vi "plotToString_MATLAB.vi"(4 "yAxisBounds":T1={"Min"={"Auto"=TRUE, "Value"=0.0}, "Max"={"Auto"=TRUE, "Value"=0.0}}, 5 "Interation number":i32, 6 "xAxisBounds":T1={"Min"={"Auto"=TRUE, "Value"=0.0}, "Max"={"Auto"=TRUE, "Value"=0.0}}, 7 "Error Bar Type":T5=enum."Standard Error", 8 "Plot Metadata":T3, 9 "Profile Number":string, 10 "Column2":dbl[](array[numeric]), 11 "Column1":dbl[](array[numeric])) -> (0 "Max Min array":dbl[][](array[numeric]), 1 "Error Bars?":bool, 2 "Data Directories":string[](array[string]), 3 "plotString":string)   [LabVIEW 2020]
uses:
  Anemometry/Anemometry Sub Vis/Data_plotting_vis/Error bar Type.ctl
  Anemometry/Anemometry Sub Vis/Data_plotting_vis/RFP_Plot_Metadata.ctl
  Anemometry/Anemometry Sub Vis/Data_plotting_vis/Error_bars_index.ctl
  Anemometry/Anemometry Sub Vis/Data_plotting_vis/gnuplotScriptComponents/minAndMax.ctl
  Anemometry/Anemometry Sub Vis/Data_plotting_vis/gnuplotScriptComponents/AutoManualNumber.ctl
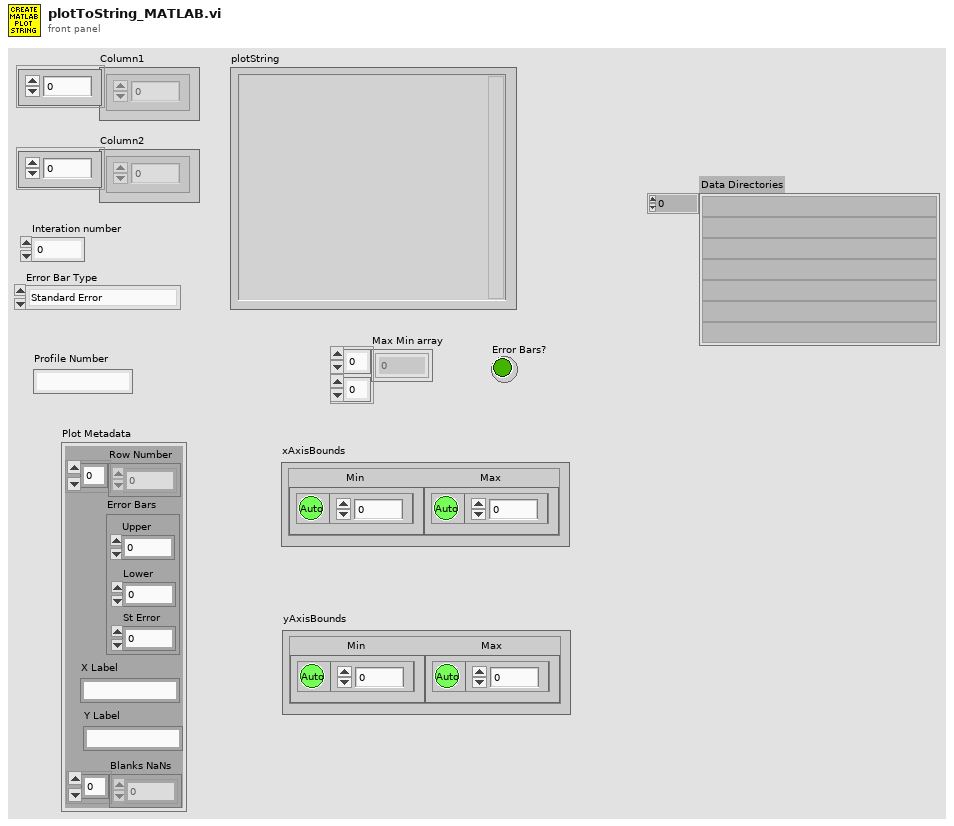
[diagram p1: front panel]
types:
  T1 = typedef "minAndMax.ctl" = cluster{"Min":T2, "Max":T2}
  T2 = typedef "AutoManualNumber.ctl" = cluster{"Auto":bool, "Value":dbl}
  T3 = typedef "RFP_Plot_Metadata.ctl" = cluster{"Row Number":i32[], "Error Bars":T4, "X Label":string, "Y Label":string, "Blanks NaNs":i32[]}
  T4 = typedef "Error_bars_index.ctl" = cluster{"Upper":i32, "Lower":i32, "St Error":i32}
  T5 = typedef "Error bar Type.ctl" = enum16{"None", "Standard Error", "Separate upper and lower"}
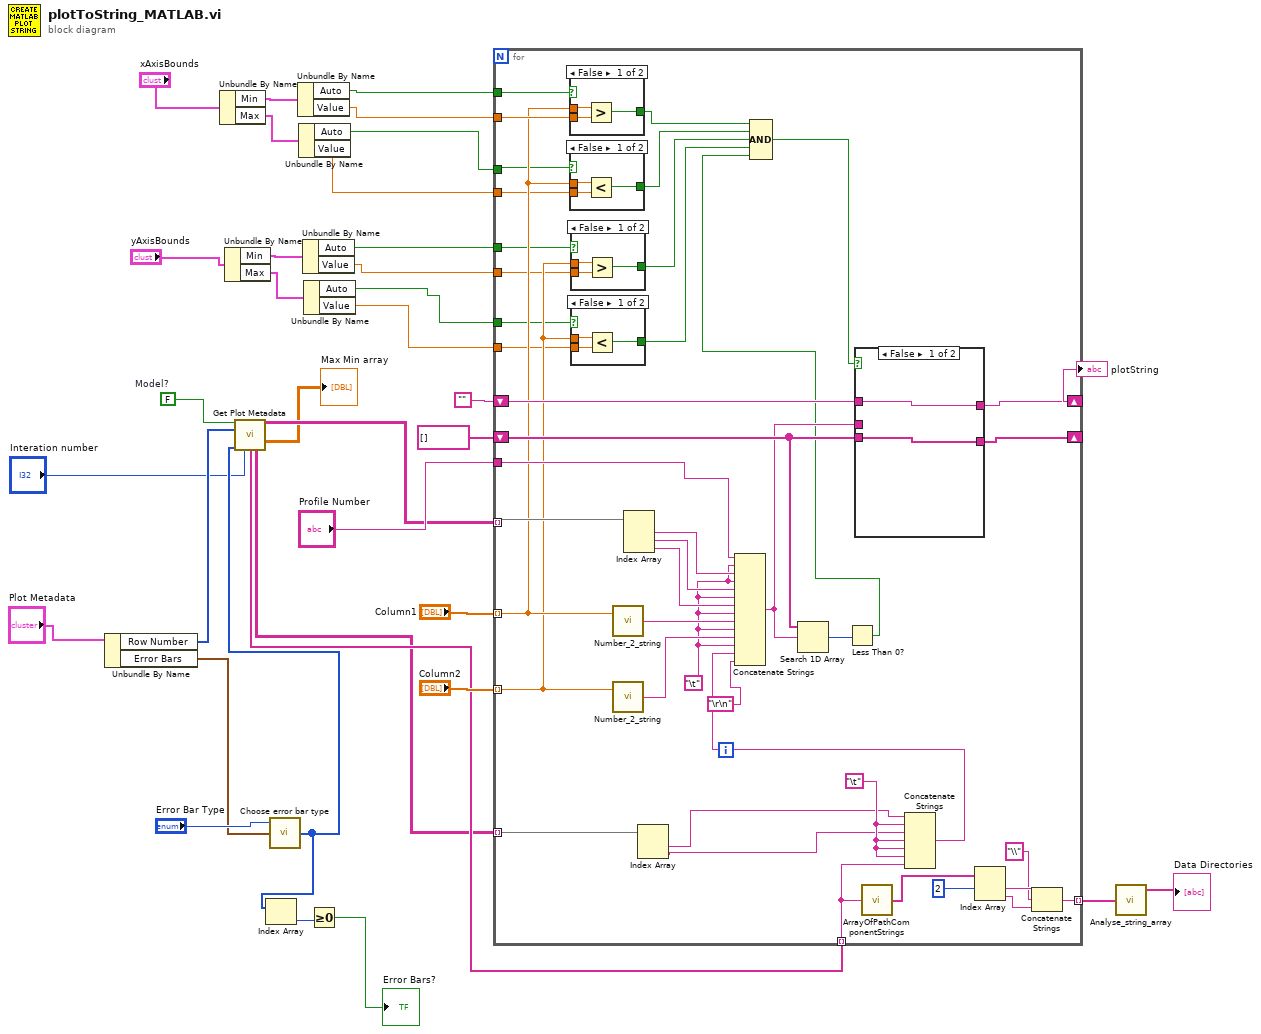
[diagram p0: block diagram]
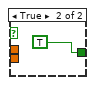
[diagram p2: hidden frame]
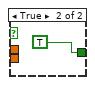
[diagram p3: hidden frame]
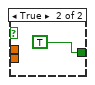
[diagram p4: hidden frame]
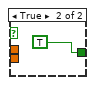
[diagram p5: hidden frame]
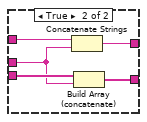
[diagram p6: hidden frame]
diagram:
  w25 = FALSE  # Model?
  n1 = Unbundle By Name("Plot Metadata") -> ("Row Number"=w28:i32[], "Error Bars"=w23:T4)
  n2 = Unbundle By Name("xAxisBounds") -> ("Min"=w16:T2, "Max"=w14:T2)
  n3 = Unbundle By Name("yAxisBounds") -> ("Min"=w9:T2, "Max"=w10:T2)
  n4 = call "Choose error bar type.vi"("Error Bars"=w23, "Error Bar Type"="Error Bar Type") -> ("Lower Upper"=w21:i32[])  [unwired: 1 in, 2 out]
  n5 = call "Get Plot Metadata.vi"("Model?"=w25, "Row Number"=w28, "Lower Upper"=w21, "Interation number"="Interation number") -> ("Lower upper"=w22:string[][], "Locations"=w27:string[][], "Max Min array"=→"Max Min array":dbl[][], "Raw Data Filenames"=w26:string[])  [unwired: 4 in, 4 out]
  n6 = Index Array(array=w21) -> (element=w20:i32)  [unwired: 1 in]
  n7 = Unbundle By Name(w16) -> ("Auto"=w15:bool, "Value"=w12:dbl)
  n8 = Unbundle By Name(w14) -> ("Auto"=w13:bool, "Value"=w11:dbl)
  n9 = Unbundle By Name(w9) -> ("Auto"=w7:bool, "Value"=w6:dbl)
  n10 = Unbundle By Name(w10) -> ("Auto"=w5:bool, "Value"=w4:dbl)
  n11 = Greater Or Equal To 0?(x=w20) -> (x >= 0?=→"Error Bars?":bool)
  n12 = for {
    tunnel: "Column1" -> [w55] mode=indexing
    shift-right: [w75] -> w31
    shift-left: "" -> [w76]
    tunnel: "Column2" -> [w51] mode=indexing
    shift-right: [w74] -> _
    shift-left: string[] [] -> [w73]
    tunnel: w27 -> [w69] mode=indexing
    tunnel: "Profile Number" -> [w64]
    tunnel: w26 -> [w42] mode=indexing
    tunnel: w22 -> [w62] mode=indexing
    tunnel: w15 -> [w58]
    tunnel: w13 -> [w53]
    tunnel: w12 -> [w56]
    tunnel: w11 -> [w54]
    tunnel: w7 -> [w50]
    tunnel: w6 -> [w49]
    tunnel: w5 -> [w48]
    tunnel: w4 -> [w47]
    tunnel: [w36] -> w3 mode=indexing
    w63 = "\t"
    w65 = "\t"
    n13 = case shown="False" w58 {
      tunnel: w56 -> [w93 _]
      tunnel: [w91 TRUE] -> w57
      tunnel: w55 -> [w92 _]
      frame False {
        n14 = Greater?(x=w92, y=w93) -> (0:w91:bool)
      }
      frame True {
      }
    }
    n15 = case shown="False" w53 {
      tunnel: w54 -> [w89 _]
      tunnel: [w87 TRUE] -> w52
      tunnel: w55 -> [w88 _]
      frame False {
        n16 = Less?(x=w88, y=w89) -> (x < y?=w87:bool)
      }
      frame True {
      }
    }
    n17 = case shown="False" w50 {
      tunnel: w49 -> [w85 _]
      tunnel: [w83 TRUE] -> w46
      tunnel: w51 -> [w84 _]
      frame False {
        n18 = Greater?(x=w84, y=w85) -> (0:w83:bool)
      }
      frame True {
      }
    }
    n19 = case shown="False" w48 {
      tunnel: w47 -> [w81 _]
      tunnel: [w79 TRUE] -> w45
      tunnel: w51 -> [w80 _]
      frame False {
        n20 = Less?(x=w80, y=w81) -> (x < y?=w79:bool)
      }
      frame True {
      }
    }
    n21 = call "Number_2_string.vi"("number"=w55) -> ("String"=w78:string)  [unwired: 1 in]
    n22 = call "Number_2_string.vi"("number"=w51) -> ("String"=w77:string)  [unwired: 1 in]
    n23 = Index Array(array=w69) -> (element #1=w66:string, element #2=w67:string, element #3=w68:string)  [unwired: 3 in]
    n24 = Index Array(array=w62) -> (element #1=w61:string, element #2=w60:string)  [unwired: 2 in]
    n25 = call "ArrayOfPathComponentStrings.vi"("PathStringIn"=w42) -> ("ArrayOfPathComponentStringsOut"=w41:string[])
    n26 = Concatenate Strings(w61, w63, w60, w63, w63, w63, w42) -> (w71:string)
    n27 = Concatenate Strings(w64, w65, w66, w65, w67, w65, w68, w65, w78, w65, w77, w65, w71, "\r\n") -> (w72:string)
    n28 = Search 1D Array(1D array=w73, element=w72) -> (index of element=w59:i32)  [unwired: 1 in]
    n29 = Less Than 0?(x=w59) -> (x < 0?=w44:bool)
    n30 = Compound Arithmetic op=AND(w57, w52, w46, w45, w44) -> (w43:bool)
    n31 = case shown="False" w43 {
      tunnel: w76 -> [w96 w101]
      tunnel: [w96 w100] -> w75
      tunnel: w72 -> [_ w97]
      tunnel: w73 -> [w95 w99]
      tunnel: [w95 w98] -> w74
      frame False {
      }
      frame True {
        n32 = Concatenate Strings(w101, w97) -> (w100:string)
        n33 = Build Array (concatenate)(w99, w97) -> (w98:string[])
      }
    }
    n34 = Index Array(array=w41, index #1=2 ("index")) -> (element #1=w39:string, element #2=w38:string)  [unwired: 1 in]
    n35 = Concatenate Strings(w39, "\\" ("string"), w38) -> (w36:string)
  }
  "plotString" <- w31
  n36 = call "Analyse_string_array.vi"("String array"=w3) -> ("Unique strings"=→"Data Directories":string[])  [unwired: 1 in, 1 out]
